vi "XIVinVout.vi"() -> ()   [LabVIEW 2018]
uses:
  <vilib>/DAQmx/write.llb/DAQmx Write (Analog DBL 1Chan 1Samp).vi
  <vilib>/DAQmx/read.llb/DAQmx Read (Analog DBL 1Chan 1Samp).vi
  <vilib>/Analysis/baseanly.llb/Mean (DBL).vi
  <vilib>/DAQmx/create/channels.llb/DAQmx Create Channel (AO-Voltage-Basic).vi
  <vilib>/DAQmx/configure/timing.llb/DAQmx Timing (Sample Clock).vi
  <vilib>/DAQmx/miscellaneous.llb/DAQmx Fill In Error Info.vi
  <vilib>/DAQmx/create/channels.llb/DAQmx Create Channel (AI-Voltage-Basic).vi
  <vilib>/Analysis/NI_AALBase.lvlib
panel:
  out "DevStd":dbl
  out "Media":dbl
  out "Waveform Chart":dbl[](graph)
  in  "sample mode 2":i32(ring)=10178 items=["Finite Samples"=10178, "Continuous Samples"=10123, "Hardware Timed Single Point"=12522]
  in  "Durata [s]":dbl=1000.0 format="%0.2f"
  in  "rate":dbl=1000.0 format="%0.2f"
  in  "canale 2":tag
  in  "input terminal configuration":i32(ring)=-1 items=["Default"=-1, "RSE"=10083, "NRSE"=10078, "Differential"=10106, "Pseudodifferential"=12529]
  in  "Time to wait":dbl
  in  "V_in (Volt)":dbl format="%0.2f"
  in  "sample mode":i32(ring)=10178 items=["Finite Samples"=10178, "Continuous Samples"=10123, "Hardware Timed Single Point"=12522]
  in  "canale":tag
  in  "output terminal configuration":i32(ring)=-1 items=["Default"=-1, "RSE"=10083, "NRSE"=10078, "Differential"=10106, "Pseudodifferential"=12529]
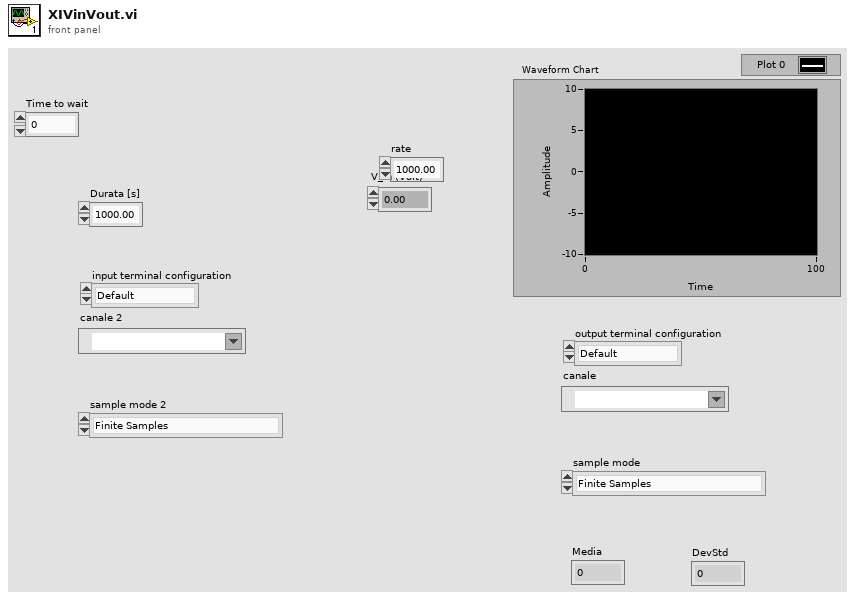
[diagram p1: front panel]
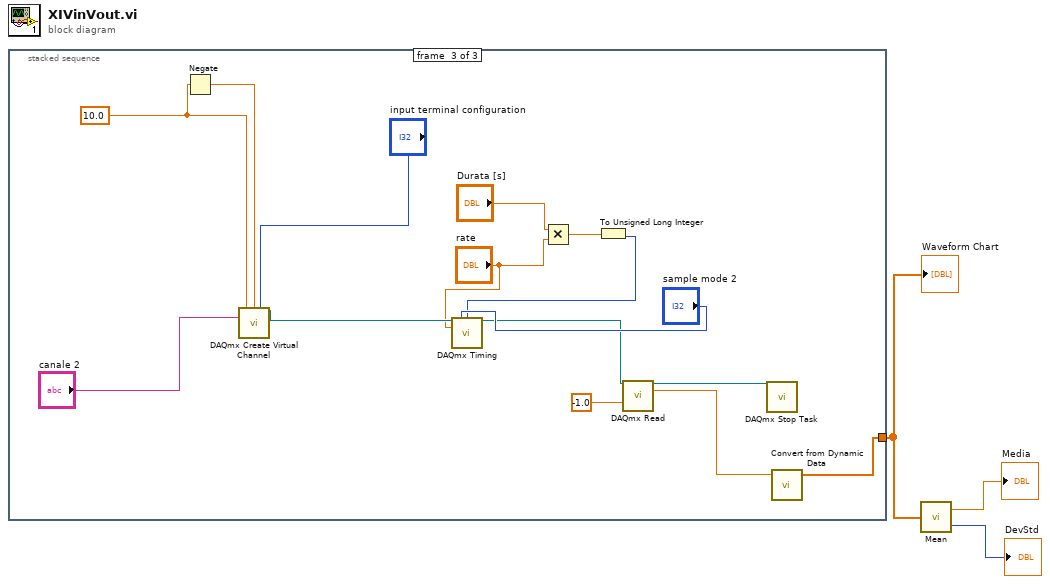
[diagram p0: block diagram]
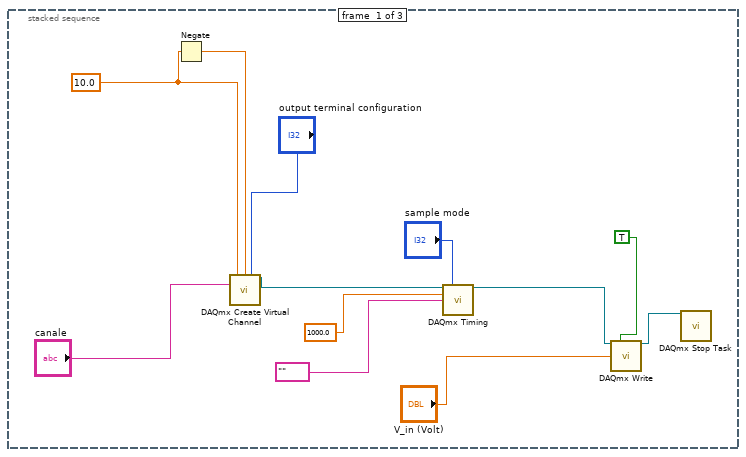
[diagram p2: hidden frame]
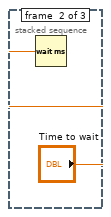
[diagram p3: hidden frame]
diagram:
  n1 = stacked-sequence {
    tunnel: [_ _ w17] -> w3
    frame #0 {
      w13 = 10.0 items=["10"=10.0, "5"=5.0, "0.5  or 1"=0.5, "0.05 or 0.2"=0.05] ("Fondo Scala")
      n2 = Negate(x=w13) -> (-x=w12:dbl)
      n3 = call-poly <vilib>:"DAQmx Create Virtual Channel.vi"("maximum value"=w13, "minimum value"=w12, "output terminal configuration"="output terminal configuration", "physical channels"="canale") -> ("task out"=w11:refnum<k21>)  [unwired: 10 in, 1 out]
      n4 = call-poly <vilib>:"DAQmx Timing.vi"("task/channels in"=w11, "sample mode"="sample mode", "rate"=1000.0, "source"=tag "") -> ("task out"=w7:refnum<k21>)  [unwired: 10 in, 1 out]
      n5 = call-poly <vilib>:"DAQmx Write.vi"("task/channels in"=w7, "auto start"=TRUE, "data"="V_in (Volt)") -> ("task out"=w6:refnum<k21>)  [unwired: 10 in, 2 out]
      n6 = call <vilib>:"DAQmx Stop Task.vi"("task/channels in"=w6) -> ()  [unwired: 13 in, 2 out]
    }
    frame #1 {
      n7 = Wait (ms)(milliseconds to wait="Time to wait") -> ()  [unwired: 1 out]
    }
    frame #2 {
      w29 = 10.0 items=["10"=10.0, "5"=5.0, "0.5  or 1"=0.5, "0.05 or 0.2"=0.05] ("Fondo Scala")
      n8 = Negate(x=w29) -> (-x=w28:dbl)
      n9 = call-poly <vilib>:"DAQmx Create Virtual Channel.vi"("maximum value"=w29, "minimum value"=w28, "input terminal configuration"="input terminal configuration", "physical channels"="canale 2") -> ("task out"=w27:refnum<k21>)  [unwired: 10 in, 1 out]
      n10 = Multiply(x="Durata [s]", y="rate") -> (x*y=w24:dbl)
      n11 = To Unsigned Long Integer(number=w24) -> (unsigned 32bit integer=w19:u32)
      n12 = call-poly <vilib>:"DAQmx Timing.vi"("task/channels in"=w27, "sample mode"="sample mode 2", "samples per channel"=w19, "rate"="rate") -> ("task out"=w22:refnum<k21>)  [unwired: 10 in, 1 out]
      n13 = call-poly <vilib>:"DAQmx Read.vi"("task/channels in"=w22, "timeout"=-1.0) -> ("task out"=w21:refnum<k21>, "data"=w18:dbl)  [unwired: 11 in, 1 out]
      n14 = call <vilib>:"DAQmx Stop Task.vi"("task/channels in"=w21) -> ()  [unwired: 13 in, 2 out]
      n15 = call "Convert from Dynamic Data"("Dynamic Data Type"=w18) -> ("Array"=w17:dbl[])  [unwired: 3 in]
    }
  }
  "Waveform Chart" <- w3
  n16 = call-poly <vilib>:"Mean.vi"("X"=w3) -> ("mean"=→"Media":dbl, "error"=→"DevStd":i32)
